vi "Client Begin Bidirectional Streaming Call.vi"(5 "Response Message Name":string, 6 "contextId":T1, 7 "Request Message Name":string, 8 "error in":errorcluster, 9 "timeout (ms)":i32=-1, 10 "Method Name":string, 11 "ClientID in":T1) -> (0 "error out":errorcluster, 2 "Call ID out":T1, 3 "ClientID out":T1)   [LabVIEW 2019, in "grpc-lvsupport.lvlib"]
uses:
  grpc-lvsupport.lvlib
  Shared/grpcId.ctl
  <vilib>/Utility/error.llb/Error Cluster From Error Code.vi
  <resource>/labview_grpc_server.dll
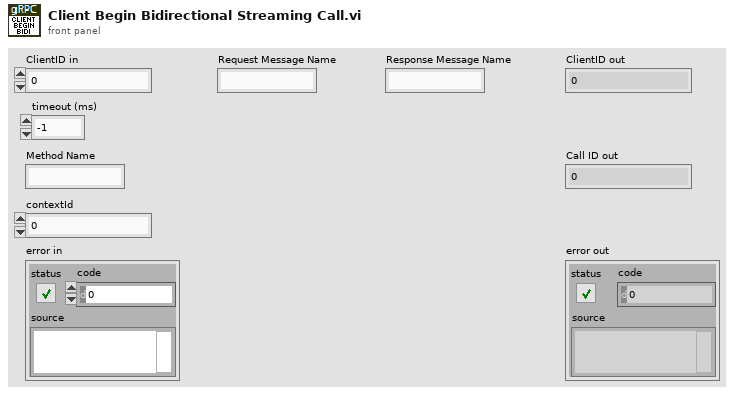
[diagram p1: front panel]
types:
  T1 = typedef "grpc-lvsupport.lvlib/grpcId.ctl" = u64
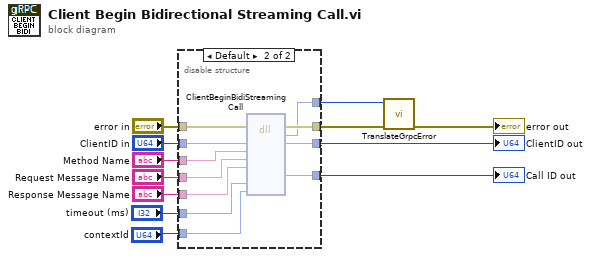
[diagram p0: block diagram]
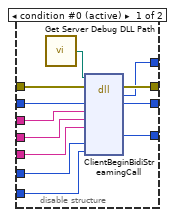
[diagram p2: hidden frame]
diagram:
  n1 = disable-structure shown="Default" {
    disable-tunnel: "error in" -> [w24 w35]
    disable-tunnel: "ClientID in" -> [w22 w34]
    disable-tunnel: [w21 w33] -> w10
    disable-tunnel: [w20 w32] -> w9
    disable-tunnel: "Method Name" -> [w19 w31]
    disable-tunnel: "Request Message Name" -> [w18 w30]
    disable-tunnel: "Response Message Name" -> [w17 w29]
    disable-tunnel: [w16 w28] -> w5
    disable-tunnel: [w15 w27] -> w3
    disable-tunnel: "timeout (ms)" -> [w14 w26]
    disable-tunnel: "contextId" -> [w13 w25]
    frame condition #0 (active) {
      n2 = call "Get Server Debug DLL Path.vi"() -> ("Server Debug DLL Path"=w23:path)
      n3 = dll-call lib="?" fn="ClientBeginBidiStreamingCall"(path in=w23, error in=w24, "ClientId"=w22, "methodName"=w19, "requestMessageName"=w18, "responseMessageName"=w17, "timeoutMs"=w14, "contextId"=w13) -> (error out=w16:errorcluster, "return type"=w15:i32, "ClientId"=w21:u64, "callId"=w20:u64)  [unwired: 7 in, 1 out]
    }
    frame condition #1 {
      n4 = dll-call lib="C:/Program Files (x86)/National Instruments/LabVIEW 2024/resource/labview_grpc_server.*" fn="ClientBeginBidiStreamingCall"(error in=w35, "ClientId"=w34, "methodName"=w31, "requestMessageName"=w30, "responseMessageName"=w29, "timeoutMs"=w26, "contextId"=w25) -> (error out=w28:errorcluster, "return type"=w27:i32, "ClientId"=w33:u64, "callId"=w32:u64)  [unwired: 8 in, 1 out]
    }
  }
  "ClientID out" <- w10
  "Call ID out" <- w9
  n5 = call "TranslateGrpcError.vi"("error in"=w5, "Error Code"=w3) -> ("error out"=→"error out":errorcluster)  [unwired: 9 in]
